vi "Scan DQMH Modules and create Maps.vi"(8 "error in":errorcluster, 9 "Include Dependencies":bool, 10 "Target Selection":string, 11 "Project":string) -> (0 "error out":errorcluster, 1 "Tree Map out":T1, 2 "map ref out":map{string, refnum<vi>}(c390), 3 "DQMH Scan Results":T2)   [LabVIEW 2019, in "Panther Dashboard.lvlib"]
doc: "Gets the Singleton and Cloneable references and creates a list of each type of DQMH Modules"
uses:
  Panther Dashboard.lvlib
  DQMH Modules Info--cluster.ctl
  Module type--enum.ctl
  Project References--cluster.ctl
  <vilib>/National Instruments/Tree Map/Tree Map Data.ctl
  <vilib>/National Instruments/Tree Map/Tree Map.lvlib
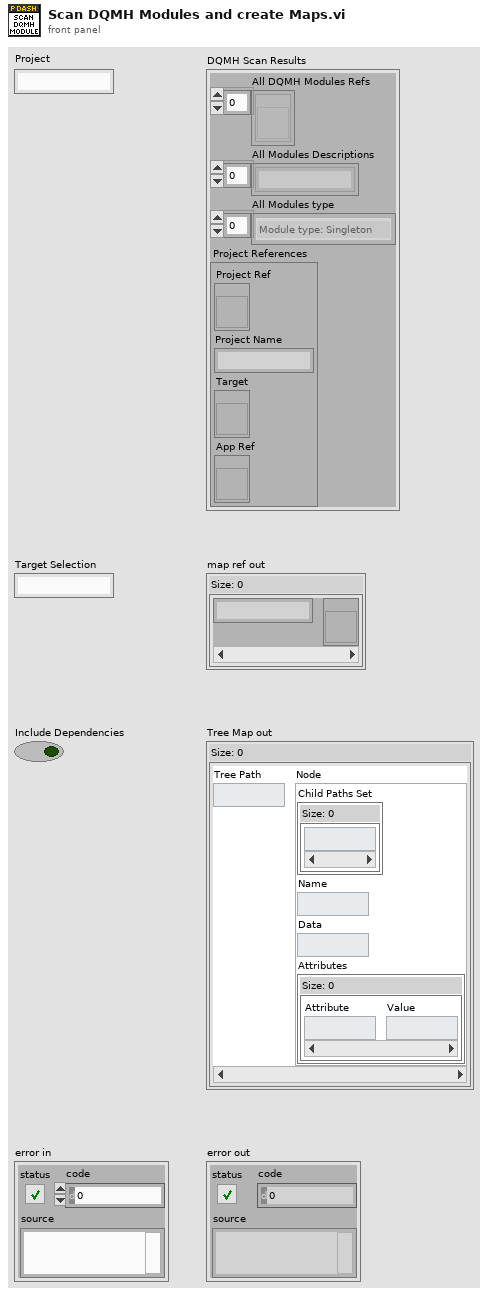
[diagram p1: front panel]
types:
  T1 = typedef "Tree Map.lvlib/Tree Map Data.ctl" = map{string, cluster{"Child Paths Set":set{string}, "Name":string, "Data":string, "Attributes":map{string, string}}}
  T2 = typedef "Panther Dashboard.lvlib/DQMH Modules Info--cluster.ctl" = cluster{"All DQMH Modules Refs":refnum<vi>[], "All Modules Descriptions":string[], "All Modules type":T3[], "Project References":T4}
  T3 = typedef "Panther Dashboard.lvlib/Module type--enum.ctl" = enum16{"Module type: Singleton", "Module type: Cloneable"}
  T4 = typedef "Panther Dashboard.lvlib/Project References--cluster.ctl" = cluster{"Project Ref":refnum<vi>, "Project Name":string, "Target":refnum<vi>, "App Ref":refnum<vi>}
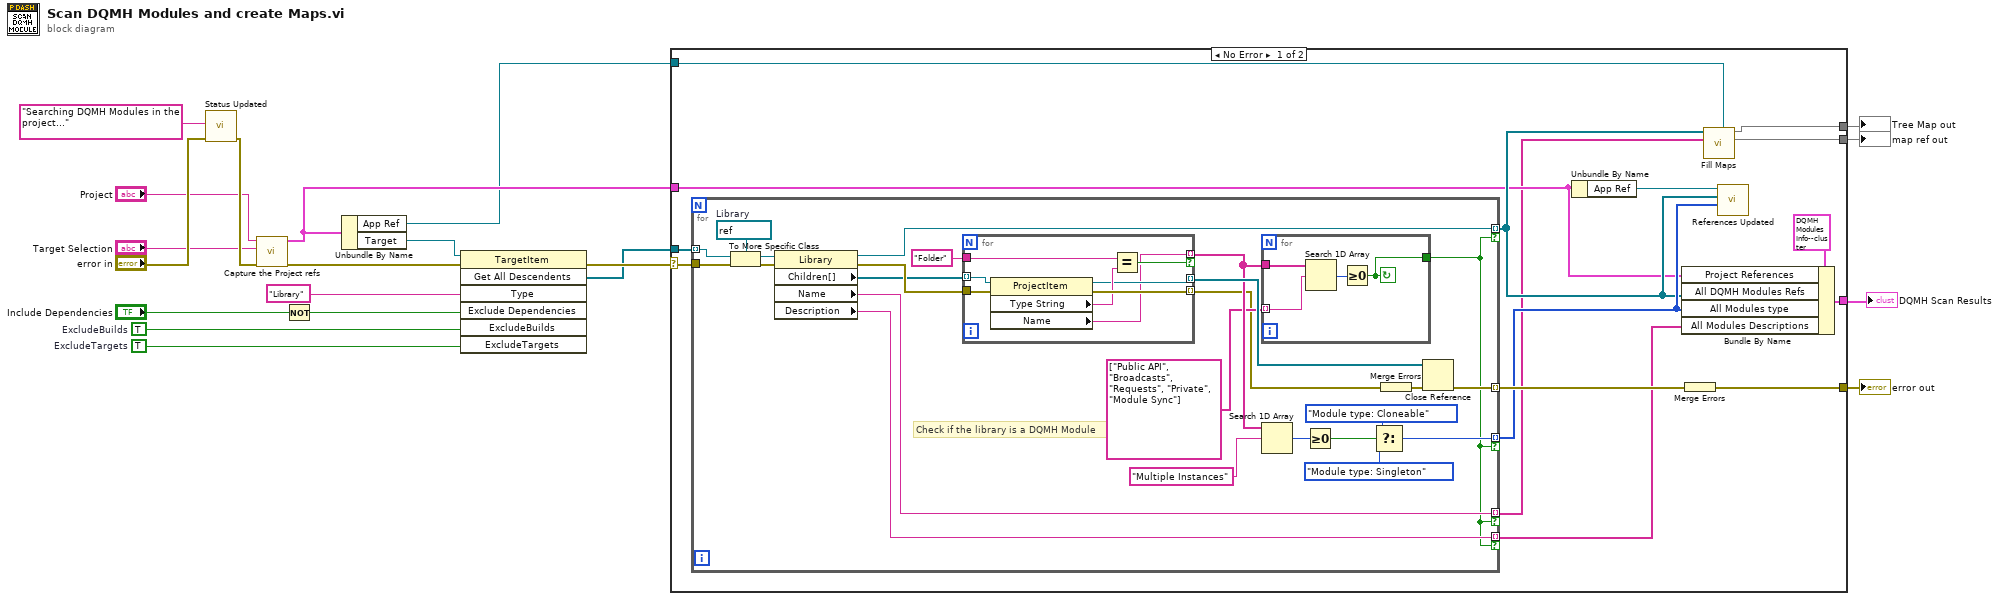
[diagram p0: block diagram]
diagram:
  w14 = TRUE  # ExcludeTargets
  w15 = TRUE  # ExcludeBuilds
  n1 = call "Status Updated.vi"("error in (no error)"="error in", "Status"="Searching DQMH Modules in the project...") -> ("error out"=w16:errorcluster)  [unwired: 9 in]
  n2 = call "Capture the Project refs.vi"("error in"=w16, "Target Selection"="Target Selection", "Project Selection"="Project") -> ("error out"=w19:errorcluster, "References"=w6:T4)  [unwired: 7 in]
  n3 = Not(x="Include Dependencies") -> (.not. x?=w10:bool)
  n4 = Unbundle By Name(w6) -> ("App Ref"=w4:refnum<vi>, "Target"=w5:refnum<vi>)
  n5 = invoke class="TargetItem" method="Get All Descendents"(reference=w5, error in=w19, "Type"="Library", "Exclude Dependencies"=w10, "ExcludeBuilds"=w15, "ExcludeTargets"=w14) -> (error out=w18:errorcluster, "All Descendents"=w7:refnum<vi>[])  [unwired: 1 in, 5 out]
  n6 = case shown="No Error" w18 {
    selector: w18 -> [w35 w72]
    tunnel: [w34 w72] -> w20
    tunnel: [w31 _] -> w11
    tunnel: w7 -> [w28 _]
    tunnel: [w30 _] -> w9
    tunnel: [w29 _] -> w8
    tunnel: w6 -> [w25 _]
    tunnel: w4 -> [w21 _]
    frame No Error {
      n7 = for {
        tunnel: [w41] -> w26 mode=indexing if=w36
        tunnel: w28 -> [w54] mode=indexing
        tunnel: [w59] -> w33 mode=indexing
        tunnel: w35 -> [w56]
        tunnel: [w53] -> w27 mode=indexing if=w36
        tunnel: [w38] -> w23 mode=indexing if=w36
        tunnel: [w37] -> w22 mode=indexing if=w36
        w39 = refnum<vi> refnum  # Library
        # "Check if the library is a DQMH Module"
        n8 = To More Specific Class(target class=w39, reference=w54, error in=w56) -> (specific class reference=w40:refnum<vi>, error out=w55:errorcluster)
        n9 = property class="Library"(reference=w40, error in=w55) -> (reference out=w41:refnum<vi>, error out=w58:errorcluster, "Children[]"=w51:refnum<vi>[], "Name"=w37:string, "Description"=w38:string)
        n10 = for {
          tunnel: [w64] -> w47 mode=indexing if=w65
          tunnel: w58 -> [w71]
          tunnel: [w70] -> w45 mode=indexing
          tunnel: [w67] -> w50 mode=indexing
          tunnel: w51 -> [w69] mode=indexing
          tunnel: "Folder" ("Type") -> [w66]
          n11 = property class="ProjectItem"(reference=w69, error in=w71) -> (reference out=w67:refnum<vi>, error out=w70:errorcluster, "Type String"=w68:string, "Name"=w64:string)
          n12 = Equal?(x=w66, y=w68) -> (x = y?=w65:bool)
        }
        n13 = for {
          tunnel: string[] ["Public API", "Broadcasts", "Requests", "Private", "Module Sync"] -> [w63] mode=indexing
          tunnel: w47 -> [w62]
          tunnel: [w60] -> w36
          stop <- w60 continue-if-true
          n14 = Search 1D Array(1D array=w62, element=w63) -> (index of element=w61:i32)  [unwired: 1 in]
          n15 = Greater Or Equal To 0?(x=w61) -> (x >= 0?=w60:bool)
        }
        n16 = Search 1D Array(1D array=w47, element="Multiple Instances") -> (index of element=w49:i32)  [unwired: 1 in]
        n17 = Greater Or Equal To 0?(x=w49) -> (x >= 0?=w44:bool)
        n18 = Select(t=Module_type--enum."Module type: Cloneable", s=w44, f=Module_type--enum."Module type: Singleton" ("Module type")) -> (s? t:f=w53:T3)
        n19 = Merge Errors(w45) -> (w57:errorcluster)
        n20 = Close Reference(reference=w50, error in (no error)=w57) -> (error out=w59:errorcluster)
      }
      n21 = Unbundle By Name(w25) -> ("App Ref"=w24:refnum<vi>)
      n22 = Bundle By Name(cluster=T2 {"All DQMH Modules Refs"=[], "All Modules Descriptions"=[], "All Modules type"=[], "Project References"={"Project Ref"=refnum, "Project Name"="", "Target"=refnum, "App Ref"=refnum}} ("DQMH Modules Info"), "Project References"=w25, "All DQMH Modules Refs"=w26, "All Modules type"=w27, "All Modules Descriptions"=w23) -> (w31:T2)
      n23 = Merge Errors(w33) -> (w34:errorcluster)
      n24 = call "Fill Maps.vi"("App Ref"=w21, "Module names"=w22, "DQMH Modules"=w26) -> ("map ref out"=w30:map{string, refnum<vi>}, "Tree Map out"=w29:T1)  [unwired: 7 in]
      n25 = call "References Updated.vi"("Modules Types"=w27, "Modules"=w26, "Application Instance"=w24) -> ()  [unwired: 8 in, 1 out]
    }
    frame Error {
    }
  }
  "error out" <- w20
  "DQMH Scan Results" <- w11
  "map ref out" <- w9
  "Tree Map out" <- w8
